vi "PH_VacuumControl.destructor.vi"(0 "i ref in":refnum<vi>, 5 "error in(no error)":errorcluster) -> (19 "error out":errorcluster)   [LabVIEW 2014, in "PH_VacuumControl.lvlib"]
doc: "This is the destructor of a class.\n\nLicense Agreement for this software:\n\nCopyright (C)\nGesellschaft für Schwerionenforschung, GSI\nPlanckstr. 1\n64291 Darmstadt\nGermany\n\nContact: D.Beck@gsi.de \n\nThis program is free software; you can redistribute it and/or modify it under the terms of the \nGNU General Public License as published by the Free Software Foundation; either version 2 of \nthe license, or (at your option) any later version.\n\nThis program is distributed in the hope that it will be useful, but WITHOUT ANY WARRANTY; \nwithout even the implied warranty of MERCHANTABILITY or FITNESS FOR A PARTICULAR PURPOSE. See the GNU General License for more details (http://www.gnu.org).\n\nGesellschaft für Schwerionenforschung, GSI\nPlanckstr. 1, 64291 Darmstadt, Germany\nFor all questions and ideas contact: M.Richter@gsi.de, H.Brand@gsi.de or D.Beck@gsi.de.\nLast update: 16-JUN-2004"
uses:
  PH_VacuumControl.lvlib
  CSlibraries-extern/DimLVEvent/LVDimInterface/LVDimInterface.lvlib
  PH_Basics/PH_PSDBWriter/PH_PSDBWriter.lvlib
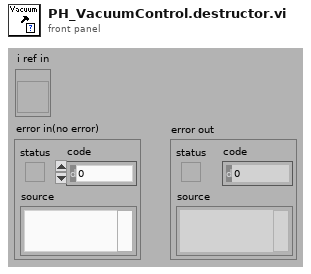
[diagram p1: front panel]
types:
  T1 = enum16{"SetAttribute", "GetAttribute", "CreateAttribute", "DestroyAttribute", "DestroyAllAtributes"}
  T2 = typedef "PH_VacuumControl.lvlib/PH_VacuumControl.i attribute.ctl" = cluster{"GUI Refs":cluster{"Exit":refnum<vi>, "Set Unit":refnum<vi>, "Device found":refnum<vi>, "Busy":refnum<vi>, "State":refnum<vi>, "Delete":refnum<vi>, "Channels":refnum<vi>, "Channel Name":refnum<vi>, "Trend":refnum<vi>, "Logarithmic":refnum<vi>, "Limit reached":refnum<vi>, "Channel Name 1 MT":refnum<vi>, "Channel Name 2 MT":refnum<vi>, "Trend MT":refnum<vi>, "Logarithmic MT":refnum<vi>, "Limit reached MT":refnum<vi>}, "Device found":bool, "Busy":bool, "Selected Unit":i32, "Channels [mbar]":T3, "Channel Names":cluster{"Channel 1":string, "Channel 2":string, "Channel 3":string, "Channel 4":string, "Channel 5":string, "Channel 6":string}, "Status":T4, "AGCxxx VISA Cluster":T5, "Instr Firmware Revision":string, "Service IDs Pressure":cluster{"Channel 1":i32, "Channel 2":i32, "Channel 3":i32, "Channel 4":i32, "Channel 5":i32, "Channel 6":i32}, "Service IDs Limits":cluster{"Channel 1":i32, "Channel 2":i32, "Channel 3":i32, "Channel 4":i32, "Channel 5":i32, "Channel 6":i32}, "Trend":cluster{"Start Point":timestamp, "Pressures [mbar] Channel 1":dbl[], "Pressures [mbar] Channel 2":dbl[], "Pressures [mbar] Channel 3":dbl[], "Pressures [mbar] Channel 4":dbl[], "Pressures [mbar] Channel 5":dbl[], "Pressures [mbar] Channel 6":dbl[], "Timebase [s]":i32[], "Trend Channel":u16, "Start Fit":dbl, "Trend Channel 1 MT":u16, "Trend Channel 2 MT":u16, "Start or continue Fit MT":dbl, "Continue or start Fit MT":dbl, "Datasets strored":i32, "Dataarray Size":i32}, "Running":bool}
  T3 = typedef "PH_VacuumControl.lvlib/PH_VacuumControl.Channels.ctl" = cluster{"Channel 1":dbl, "Channel 2":dbl, "Channel 3":dbl, "Channel 4":dbl, "Channel 5":dbl, "Channel 6":dbl, "Name Channel 1":string, "Name Channel 2":string, "Name Channel 3":string, "Name Channel 4":string, "Name Channel 5":string, "Name Channel 6":string, "Upper Limit":dbl, "Upper Limit 2":dbl, "Upper Limit 3":dbl, "Upper Limit 4":dbl, "Upper Limit 5":dbl, "Upper Limit 6":dbl}
  T4 = typedef "PH_StatusHandler.lvlib/PH_StatusHandler.Status.ctl" = i16
  T5 = typedef "AGCxxx - Driver.lvlib/AGCxxx VISA Control.ctl" = cluster{"VISA resource name":refnum<visa-resource-name>, "VISA Timeout Value (1000 ms)":u32, "Lock Timeout (1000 ms)":u32, "MAX Channel (6)":i32}
  T6 = cluster{"Channel 1":i32, "Channel 2":i32, "Channel 3":i32, "Channel 4":i32, "Channel 5":i32, "Channel 6":i32}
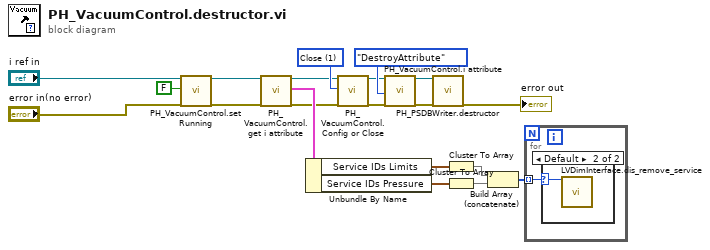
[diagram p0: block diagram]
diagram:
  w15 = u16 1 items=["Configure", "Close"] ("Action")
  n1 = call "PH_VacuumControl.set Running.vi"("VI in"="i ref in", "Running"=FALSE, "error in (no error)"="error in(no error)") -> ("VI out"=w2:refnum<vi>, "error out"=w4:errorcluster)  [unwired: 15 in]
  n2 = call "PH_VacuumControl.get i attribute.vi"("i ref in"=w2, "error in (no error)"=w4) -> ("i ref out"=w6:refnum<vi>, "i attribute"=w14:T2, "error out"=w7:errorcluster)  [unwired: 15 in]
  n3 = Unbundle By Name(w14) -> ("Service IDs Limits"=w9:T6, "Service IDs Pressure"=w12:T6)
  n4 = call "PH_VacuumControl.Config or Close.vi"("i ref in"=w6, "Action"=w15, "error in (no error)"=w7) -> ("i ref out"=w16:refnum<vi>, "error out"=w17:errorcluster)  [unwired: 15 in]
  n5 = call "PH_VacuumControl.i attribute.vi"("VI Refnum"=w16, "Action"=T1."DestroyAttribute", "error in (no error)"=w17) -> ("VI Refnum out"=w18:refnum<vi>, "error out"=w19:errorcluster)  [unwired: 14 in, 1 out]
  n6 = call "PH_PSDBWriter.destructor.vi"("i ref in"=w18, "error in(no error)"=w19) -> ("error out"=→"error out":errorcluster)  [unwired: 17 in]
  n7 = Cluster To Array(cluster=w9) -> (array=w8:i32[])
  n8 = Cluster To Array(cluster=w12) -> (array=w11:i32[])
  n9 = Build Array (concatenate)(w8, w11) -> (w10:i32[])
  n10 = for {
    tunnel: w10 -> [w21] mode=indexing
    n11 = case shown="Default" w21 {
      selector: w21 -> [_ w22]
      frame -1 {
      }
      frame Default {
        n12 = call "LVDimInterface.dis_remove_service.vi"("my_serviceID"=w22) -> ()  [unwired: 18 in, 1 out]
      }
    }
  }
